vi "GetServerNiceName.vi"(0 "ROS":T1={"topic port"=0, "Node"="", "topic"="", "type"="", "node port"=0, "error "={"status"=FALSE, "code"=0, "source"=""}, "Direction"=enum."Node", "Update (ms)"=1, "FIFO size"=0}, 1 "Text to add":string) -> (2 "String":string)   [LabVIEW 2016]
doc: "Gets server name"
uses:
  _ROSControl.ctl
  _ROSDirection.ctl
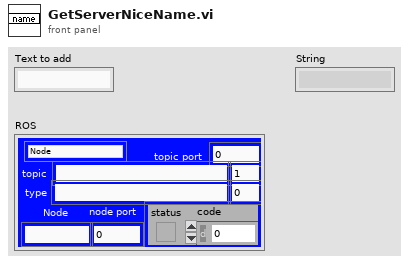
[diagram p1: front panel]
types:
  T1 = typedef "_ROSControl.ctl" = cluster{"topic port":u16, "Node":string, "topic":string, "type":string, "node port":u16, "error ":errorcluster, "Direction":T2, "Update (ms)":u16, "FIFO size":u16}
  T2 = typedef "_ROSDirection.ctl" = enum16{"Node", "Publisher", "Subscriber", "ServiceClient", "ServiceProvider"}
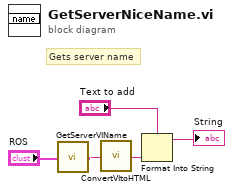
[diagram p0: block diagram]
diagram:
  # "Gets server name"
  n1 = call "GetServerVIName.vi"("ROS"="ROS") -> ("vi name"=w3:string)
  n2 = call "ConvertVItoHTML.vi"("vi name"=w3) -> ("Server Name"=w5:string)  [unwired: 1 out]
  n3 = Format Into String(format string="Text to add", w5) -> (resulting string=→"String":string)  [unwired: 2 in, 1 out]
